vi "ble_connect_to_device.vi"(1 "Address Type":T1=1 items=["Public", "Random"], 5 "Connection Interval Max (95ms)":u16=95, 6 "Latency(0)":u16, 7 "Connection Interval Min (75ms)":u16=75, 8 "error in (no error)":errorcluster, 9 "Timeout(1000ms)":u16=1000, 10 "MAC Address":string, 11 "COM Bluegiga in":refnum<visa-resource-name>) -> (0 "error out":errorcluster, 3 "COM Bluegiga out":refnum<visa-resource-name>, 4 "Connection Status":T2={"MAC Address"="", "cnx handle"=0, "cnx flags"=0, "Address Type"=125, "Connection Interval (ms)"=125, "Timeout(ms)"=125, "Latency"=0, "bonding handle"=0} {"Address Type" items=["Public", "Random"]})   [LabVIEW 2015]
uses:
  type_def/connection_status_bundle.ctl
  type_def/address_type.ctl
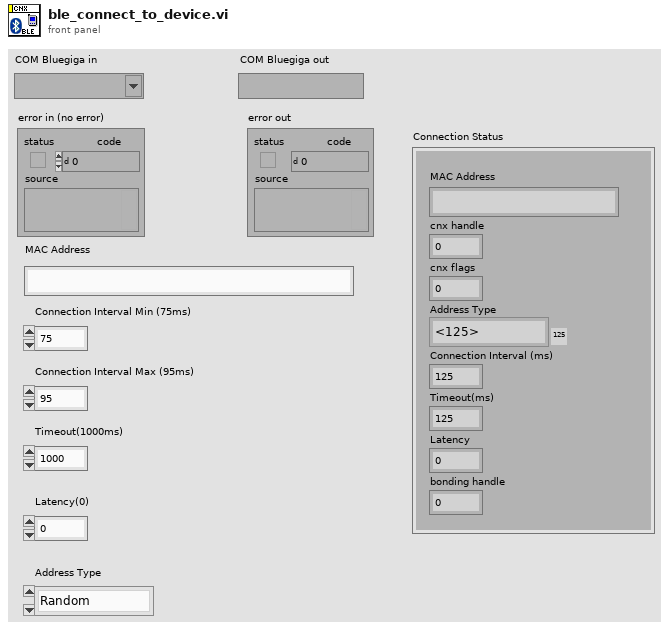
[diagram p1: front panel]
types:
  T1 = typedef "address_type.ctl" = u8
  T2 = typedef "connection_status_bundle.ctl" = cluster{"MAC Address":string, "cnx handle":u8, "cnx flags":u8, "Address Type":T1, "Connection Interval (ms)":u16, "Timeout(ms)":u16, "Latency":u16, "bonding handle":u8}
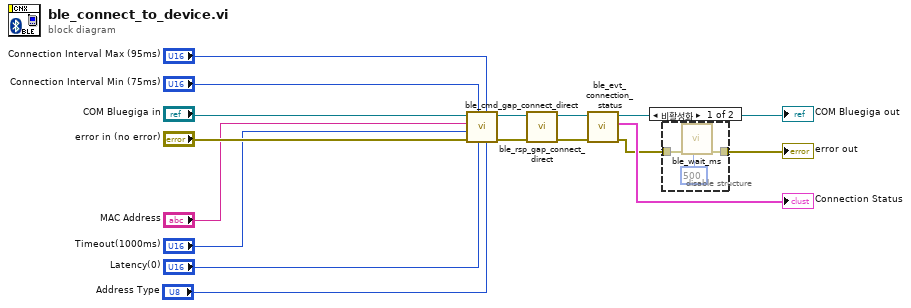
[diagram p0: block diagram]
diagram:
  n1 = call "ble_cmd_gap_connect_direct.vi"("Address Type"="Address Type", "Connection Interval Max (95ms)"="Connection Interval Max (95ms)", "Latency(0)"="Latency(0)", "Connection Interval Min (75ms)"="Connection Interval Min (75ms)", "error in (no error)"="error in (no error)", "Timeout(1000ms)"="Timeout(1000ms)", "MAC Address"="MAC Address", "COM Bluegiga in"="COM Bluegiga in") -> ("error out"=w14:errorcluster, "COM Bluegiga out"=w13:refnum<visa-resource-name>)  [unwired: 2 in]
  n2 = call "ble_rsp_gap_connect_direct.vi"("error in (no error)"=w14, "COM Bluegiga in"=w13) -> ("error out"=w4:errorcluster, "COM Bluegiga out"=w5:refnum<visa-resource-name>)  [unwired: 7 in, 1 out]
  n3 = call "ble_evt_connection_status.vi"("error in (no error)"=w4, "COM Bluegiga in"=w5) -> ("error out"=w2:errorcluster, "Connection Status"=→"Connection Status":T2, "COM Bluegiga out"=→"COM Bluegiga out":refnum<visa-resource-name>)  [unwired: 7 in]
  n4 = disable-structure shown="비활성화" {
    disable-tunnel: w2 -> [w19 w20]
    disable-tunnel: [w18 w20] -> w1
    frame Disabled {
      n5 = call "ble_wait_ms.vi"("milliseconds to wait (100)"=u32 500, "error in (no error)"=w19) -> ("error out"=w18:errorcluster)  [unwired: 9 in]
    }
    frame Enabled {
    }
  }
  "error out" <- w1
